vi "Queue Reference (library variable).vi"() -> ()   [LabVIEW 2016, in "Error Manager.lvlib" / "Error Window Loop Queue.lvclass"]
uses:
  Error Window Loop Queue.lvclass
  Command (enum).ctl
  Message (cluster).ctl
panel:
  in  "Queue Reference":refnum<queue>
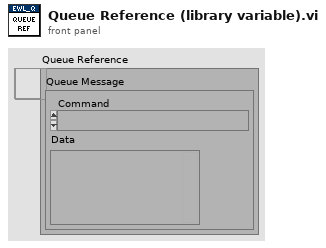
[diagram p1: front panel]
diagram:
